vi "ingest_mcapProtobufTimeseries.vi"(6 "Channel Filter":refnum<class "channelFilter.lvclass">, 8 "error in":errorcluster, 9 "Target":refnum<class "target.lvclass">, 10 "Source":refnum<class "source.lvclass">, 11 "Nominal Client in":refnum<class "Nominal Client.lvclass">) -> (0 "error out":errorcluster, 1 "datasetRid":string, 2 "datasetFileId":string, 3 "Nominal Client out":refnum<class "Nominal Client.lvclass">)   [LabVIEW 2020, in "Nominal Client.lvclass"]
doc: "Triggers an ingest job, allowing either creating a new dataset or uploading to an existing one. This endpoint is meant to supersede all other ingestion endpoints as their functionality gets migrated to this one."
uses:
  Nominal Client.lvclass
  datasources/target/target.lvclass
  datasources/source/source.lvclass
  nominal types/channelFilter/channelFilter.lvclass
  ts.logtime/ts.logtime.lvclass
  Nominal Client.lvclass/Nominal Client.ctl
  datasources/target/target.lvclass/target.ctl
  4690b3d5-22f0-4aee-9331-ce368bb25e7c.vi
  datasources/target/workspace.set.vi
  <vilib>/JDP Science/JSONtext/support/Format JSON Object.vi
  <vilib>/JDP Science/JSONtext/JSON text to Variant.vi
  <vilib>/JDP Science/JSONtext/LVClass Serializer/JSONtext LVClass Serializer.lvclass
  <vilib>/JDP Science/JSONtext/JSONtext.lvlib
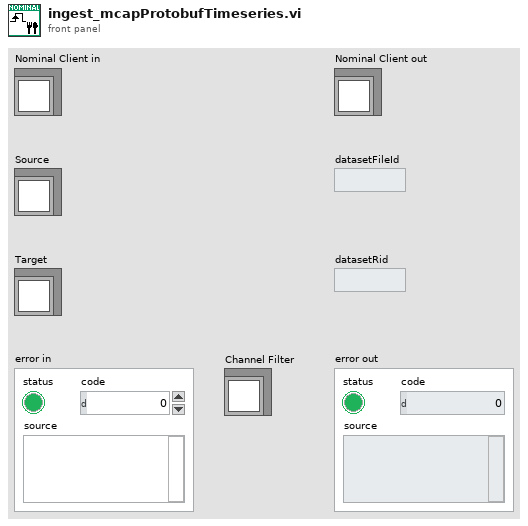
[diagram p1: front panel]
types:
  T1 = cluster{"type":string, "dataset":cluster{"datasetFileId":string, "datasetRid":string}}
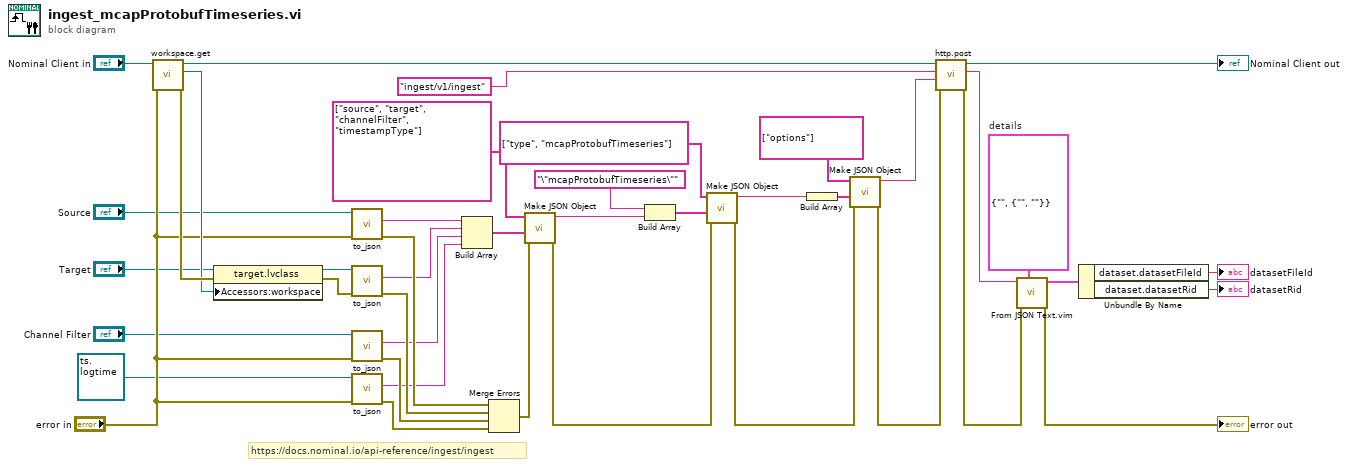
[diagram p0: block diagram]
diagram:
  w13 = T1 {"type"="", "dataset"={"datasetFileId"="", "datasetRid"=""}}  # details
  # "https://docs.nominal.io/api-reference/ingest/ingest"
  n1 = call "workspace.get.vi"("error in"="error in", "Nominal Client in"="Nominal Client in") -> ("error out"=w42:errorcluster, "workspace"=w30:refnum<class "workspace.lvclass">, "Nominal Client out"=w28:refnum<class "Nominal Client.lvclass">)  [unwired: 7 in]
  n2 = property class="target.lvclass"(reference="Target", error in=w42, "Accessors:workspace"=w30) -> (reference out=w31:refnum<class "target.lvclass">, error out=w32:errorcluster)
  n3 = call-dynamic "to_json.vi"("error in"="error in", "source in"="Source") -> ("error out"=w36:errorcluster, "json"=w39:string)  [unwired: 6 in, 2 out]
  n4 = call-dynamic "to_json.vi"("error in"=w32, "target in"=w31) -> ("error out"=w35:errorcluster, "json"=w33:string)  [unwired: 6 in, 2 out]
  n5 = call-dynamic "to_json.vi"("error in"="error in", "channelFilter in"="Channel Filter") -> ("error out"=w27:errorcluster, "json"=w23:string)  [unwired: 6 in, 2 out]
  n6 = call-dynamic "to_json.vi"("error in"="error in", "ts.logtime in"=refnum<class "ts.logtime.lvclass"> refnum ("ts.logtime.lvclass")) -> ("error out"=w26:errorcluster, "json"=w22:string)  [unwired: 6 in, 2 out]
  n7 = Build Array(w39, w33, w23, w22) -> (w37:string[])
  n8 = Merge Errors(w36, w35, w27, w26) -> (w34:errorcluster)
  n9 = call <vilib>:"Make JSON Object.vi"("error in (no error)"=w34, "JSON Items"=w37, "Item Names"=string[] ["source", "target", "channelFilter", "timestampType"] ("Path")) -> ("error out"=w14:errorcluster, "<JSON>"=w15:string)  [unwired: 7 in]
  n10 = Build Array("\"mcapProtobufTimeseries\"" ("JSON"), w15) -> (w17:string[])
  n11 = call <vilib>:"Make JSON Object.vi"("error in (no error)"=w14, "JSON Items"=w17, "Item Names"=string[] ["type", "mcapProtobufTimeseries"] ("JSON")) -> ("error out"=w1:errorcluster, "<JSON>"=w6:string)  [unwired: 7 in]
  n12 = Build Array(w6) -> (w5:string[])
  n13 = call <vilib>:"Make JSON Object.vi"("error in (no error)"=w1, "JSON Items"=w5, "Item Names"=string[] ["options"] ("JSON")) -> ("error out"=w2:errorcluster, "<JSON>"=w3:string)  [unwired: 7 in]
  n14 = call "http.post.vi"("error in"=w2, "Request body"=w3, "Path"="ingest/v1/ingest", "Nominal Client in"=w28) -> ("error out"=w8:errorcluster, "Response"=w9:string, "Nominal Client out"=→"Nominal Client out":refnum<class "Nominal Client.lvclass">)  [unwired: 4 in, 1 out]
  n15 = call "From JSON Text.vim"("Data Type and Default Value"=w13, "error in (no error)"=w8, "JSON"=w9) -> ("error out"=→"error out":errorcluster, "Data out"=w12:T1)  [unwired: 7 in]
  n16 = Unbundle By Name(w12) -> ("dataset.datasetFileId"=→"datasetFileId":string, "dataset.datasetRid"=→"datasetRid":string)
